vi "getVariaReadings.vi"(8 "error in (no error)":errorcluster, 11 "COMport":string="COM6") -> (0 "error out":errorcluster, 2 "monitorInputPercent":dbl)   [LabVIEW 2015]
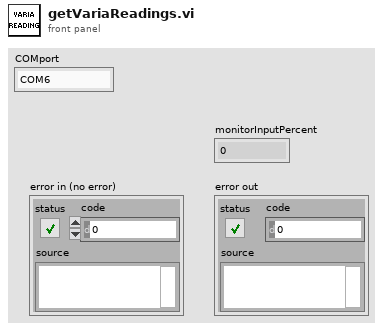
[diagram p1: front panel]
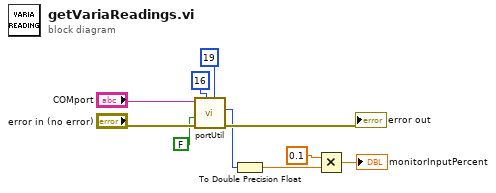
[diagram p0: block diagram]
diagram:
  n1 = call "portUtil.vi"("Register"=u8 19, "Destination"=u8 16, "error in (no error)"="error in (no error)", "WriteNotRead"=FALSE, "COMport"="COMport") -> ("error out"=→"error out":errorcluster, "Long"=w6:i32)  [unwired: 4 in, 1 out]
  n2 = To Double Precision Float(number=w6) -> (double precision float=w3:dbl)
  n3 = Multiply(x=0.1, y=w3) -> (x*y=→"monitorInputPercent":dbl)
